vi "BuildWiFiPython.vi"(9 "SystemLink":T1={"APIKey"="", "Tag"="", "Type"="STRING"}, 11 "WiFi":cluster{"SSID":string, "Key":string}) -> (1 "Repeated call":string, 2 "Setup":string, 3 "Headers":string)   [LabVIEW 2016]
panel:
  out "URL":string
  out "Value URL":string
  in  "Tag":string
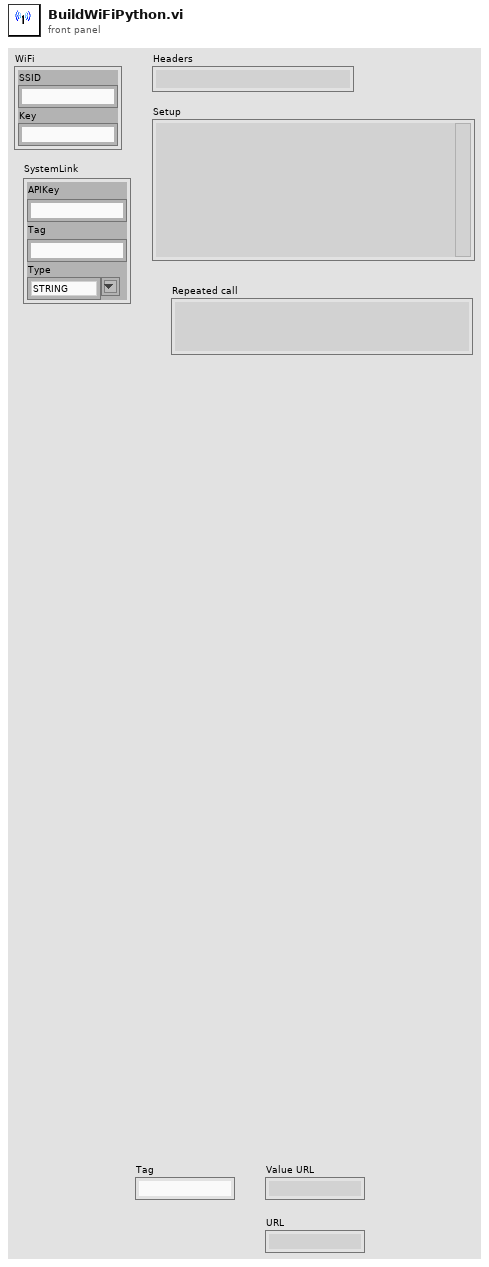
[diagram p1: front panel]
types:
  T1 = cluster{"APIKey":string, "Tag":string, "Type":string}
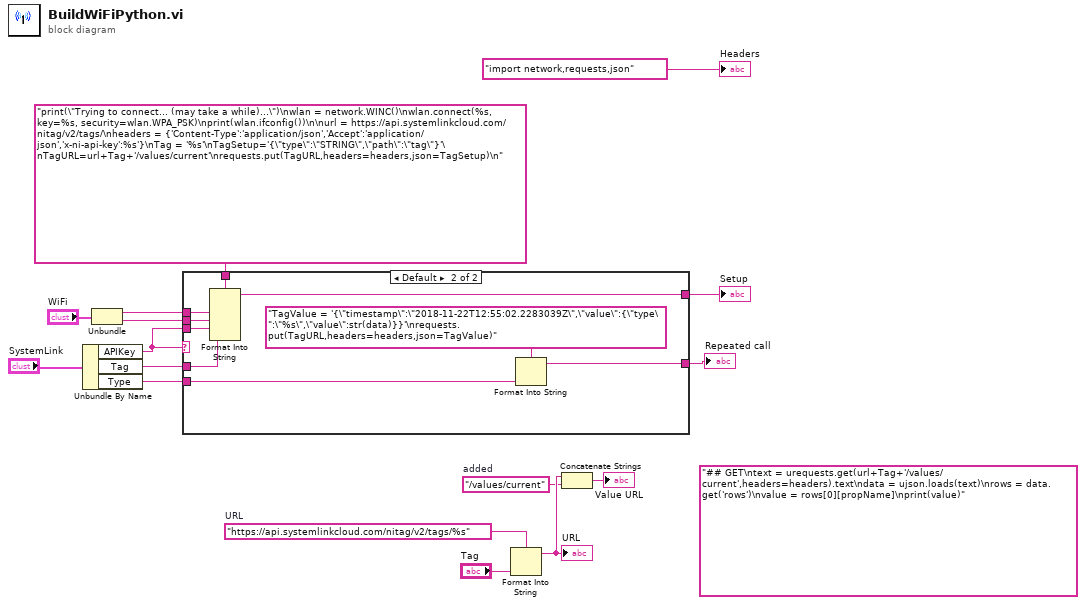
[diagram p0: block diagram]
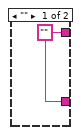
[diagram p2: hidden frame]
diagram:
  (unwired) "## GET\ntext = urequests.get(url+Tag+'/values/current',headers=headers).text\ndata = ujson.loads(text)\nrows = data.get('rows')\nvalue = rows[0][propName]\nprint(value)"
  w7 = "/values/current"  # added
  w6 = "https://api.systemlinkcloud.com/nitag/v2/tags/%s"  # URL
  n1 = Unbundle By Name("SystemLink") -> ("APIKey"=w1:string, "Tag"=w4:string, "Type"=w3:string)
  n2 = Unbundle("WiFi") -> ("SSID"=w13:string, "Key"=w14:string)
  n3 = case shown="Default" w1 {
    tunnel: [w17 w26] -> w15
    tunnel: w14 -> [_ w25]
    tunnel: w13 -> [_ w24]
    tunnel: "print(\"Trying to connect... (may take a while)...\")\nwlan = network.WINC()\nwlan.connect(%s, key=%s, security=wlan.WPA_PSK)\nprint(wlan.ifconfig())\n\nurl = https://api.systemlinkcloud.com/nitag/v2/tags/\nheaders = {'Content-Type':'application/json','Accept':'application/json','x-ni-api-key':%s'}\nTag = '%s'\nTagSetup='{\"type\":\"STRING\",\"path\":\"tag\"}'\nTagURL=url+Tag+'/values/current'\nrequests.put(TagURL,headers=headers,json=TagSetup)\n" -> [_ w23]
    tunnel: w1 -> [_ w22]
    tunnel: w4 -> [_ w21]
    tunnel: w3 -> [_ w20]
    tunnel: [w17 w18] -> w2
    frame "" {
      w17 = ""
    }
    frame Default {
      n4 = Format Into String(format string=w23, w24, w25, w22, w21) -> (resulting string=w26:string)  [unwired: 2 in, 1 out]
      n5 = Format Into String(format string="TagValue = '{\"timestamp\":\"2018-11-22T12:55:02.2283039Z\",\"value\":{\"type\":\"%s\",\"value\":str(data)}}'\nrequests.put(TagURL,headers=headers,json=TagValue)", w20) -> (resulting string=w18:string)  [unwired: 2 in, 1 out]
    }
  }
  "Setup" <- w15
  "Repeated call" <- w2
  n6 = Format Into String(format string=w6, "Tag") -> (resulting string=w8:string)  [unwired: 2 in, 1 out]
  "URL" <- w8
  n7 = Concatenate Strings(w8, w7) -> (→"Value URL":string)
  "Headers" <- "import network,requests,json"
